vi "Select state based on Error.vi"(8 "error in (no error)":errorcluster, 11 "Wanted state":T1) -> (3 "Next State":T1)   [LabVIEW 2023]
uses:
  System states.ctl
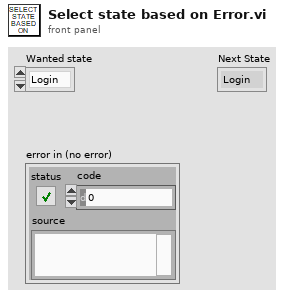
[diagram p1: front panel]
types:
  T1 = typedef "System states.ctl" = enum16{"Login", "Initialize", "Idle", "Erasing", "Connect relays", "Disconnect relays", "Deinitialize", "Set variables"}
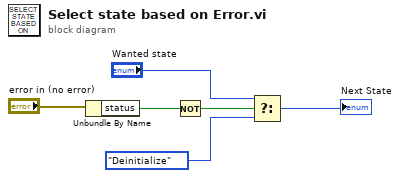
[diagram p0: block diagram]
diagram:
  n1 = Unbundle By Name("error in (no error)") -> ("status"=w2:bool)
  n2 = Not(x=w2) -> (.not. x?=w1:bool)
  n3 = Select(t="Wanted state", s=w1, f=System_states."Deinitialize") -> (s? t:f=→"Next State":T1)
